vi "sysparam.vi"() -> (1 "C":dbl[][](array[numeric]), 2 "K":dbl[][](array[numeric]), 3 "A":dbl[][](array[numeric]))   [LabVIEW 2015]
uses:
  <vilib>/imath/engines/lvmath2/RunTimeEngine/NodeEndStatement/NIMS_NodeEndStatement_Output.vi
  <instcachedir>/0/NIMS_NodeEndStatement_Output_53EC0D466D134D7ABD903AC30B43404B.lvgen/NIMS_NodeEndStatement_Output_53EC0D466D134D7ABD903AC30B43404B_010.vi
  <instcachedir>/0/NIMS_NodeEndStatement_Output_53EC0D466D134D7ABD903AC30B43404B.lvgen/NIMS_NodeEndStatement_Output_53EC0D466D134D7ABD903AC30B43404B_002.vi
  <vilib>/imath/engines/lvmath2/RunTimeEngine/ErrorHandling/NIMS_Finalize Error.vi
panel:
  in  "az":dbl=0.45
  in  "ay":dbl=0.45
  in  "ax":dbl=0.45
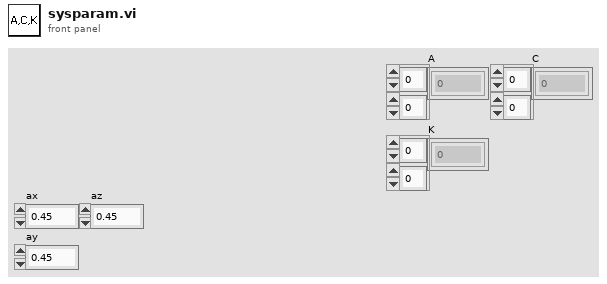
[diagram p1: front panel]
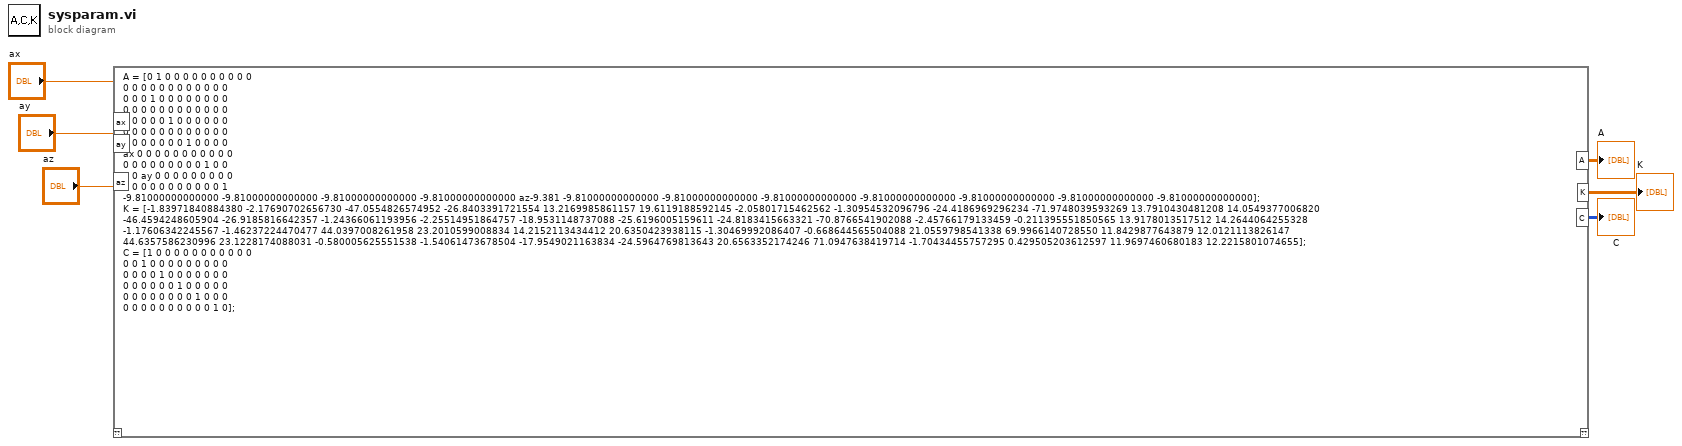
[diagram p0: block diagram]
diagram:
  n1 = mathscript code="A = [0\t1\t0\t0\t0\t0\t0\t0\t0\t0\t0\t0\n0\t0\t0\t0\t0\t0\t0\t0\t0\t0\t0\t0\n0\t0\t0\t1\t0\t0\t0\t0\t0\t0\t0\t0\n0\t0\t0\t0\t0\t0\t0\t0\t0\t0\t0\t0\n0\t0\t0\t0\t0\t1\t0\t0\t0\t0\t0\t0\n0\t0\t0\t0\t0\t0\t0\t0\t0\t0\t0\t0\n0\t0\t0\t0\t0\t0\t0\t1\t0\t0\t0\t0\nax\t0\t0\t0\t0\t0\t0\t0\t0\t0\t0\t0\n0\t0\t0\t0\t0\t0\t0\t0\t0\t1\t0\t0\n0\t0\tay\t0\t0\t0\t0\t0\t0\t0\t0\t0\n0\t0\t0\t0\t0\t0\t0\t0\t0\t0\t0\t1\n-9.81000000000000\t-9.81000000000000\t-9.81000000000000\t-9.81000000000000\taz-9.381\t-9.81000000000000\t-9.81000000000000\t-9.81000000000000\t-9.81000000000000\t-9.81000000000000\t-9.81000000000000\t-9.81000000000000];\nK = [-1.83971840884380\t-2.17690702656730\t-47.0554826574952\t-26.8403391721554\t13.2169985861157\t19.6119188592145\t-2.05801715462562\t-1.30954532096796\t-24.4186969296234\t-71.9748039593269\t13.7910430481208\t14.0549377006820\n-46.4594248605904\t-26.9185816642357\t-1.24366061193956\t-2.25514951864757\t-18.9531148737088\t-25.6196005159611\t-24.8183415663321\t-70.8766541902088\t-2.45766179133459\t-0.211395551850565\t13.9178013517512\t14.2644064255328\n-1.17606342245567\t-1.46237224470477\t44.0397008261958\t23.2010599008834\t14.2152113434412\t20.6350423938115\t-1.30469992086407\t-0.668644565504088\t21.0559798541338\t69.9966140728550\t11.8429877643879\t12.0121113826147\n44.6357586230996\t23.1228174088031\t-0.580005625551538\t-1.54061473678504\t-17.9549021163834\t-24.5964769813643\t20.6563352174246\t71.0947638419714\t-1.70434455757295\t0.429505203612597\t11.9697460680183\t12.2215801074655];\nC = [1\t0\t0\t0\t0\t0\t0\t0\t0\t0\t0\t0\n0\t0\t1\t0\t0\t0\t0\t0\t0\t0\t0\t0\n0\t0\t0\t0\t1\t0\t0\t0\t0\t0\t0\t0\n0\t0\t0\t0\t0\t0\t1\t0\t0\t0\t0\t0\n0\t0\t0\t0\t0\t0\t0\t0\t1\t0\t0\t0\n0\t0\t0\t0\t0\t0\t0\t0\t0\t0\t1\t0];"("ax"="ax", "ay"="ay", "az"="az") -> ("A"=→"A":dbl[][], "K"=→"K":dbl[][], "C"=→"C":i32[][])  [unwired: 1 in, 1 out]
